vi "Function_queue receiver.vi"(8 "error in (no error)":errorcluster, 9 "Clone Name":string, 11 "Queue in":refnum<queue>) -> (0 "error out":errorcluster, 1 "Filename":string, 3 "Queue out":refnum<queue>, 4 "message":string, 5 "Stop":bool)   [LabVIEW 2022 SP3]
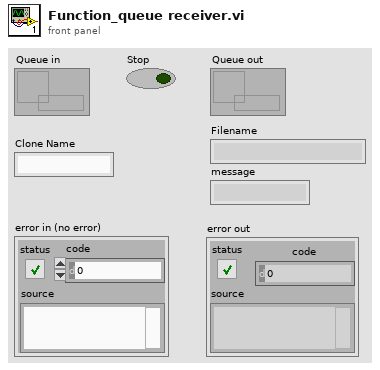
[diagram p1: front panel]
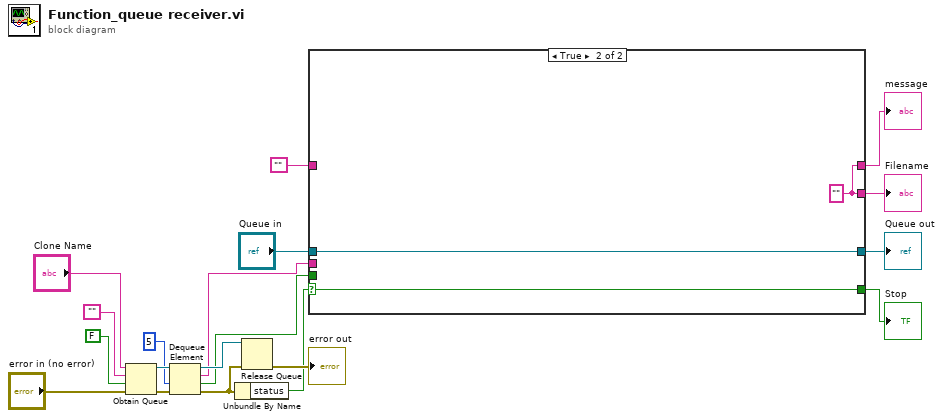
[diagram p0: block diagram]
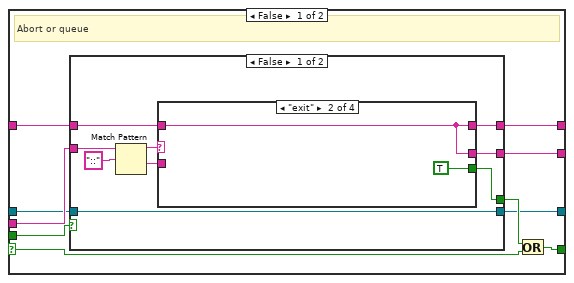
[diagram p2: hidden frame]
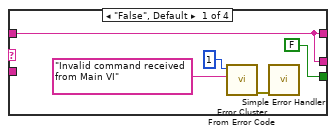
[diagram p3: hidden frame]
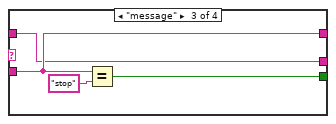
[diagram p4: hidden frame]
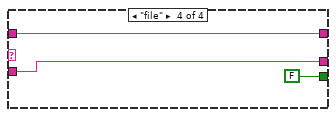
[diagram p5: hidden frame]
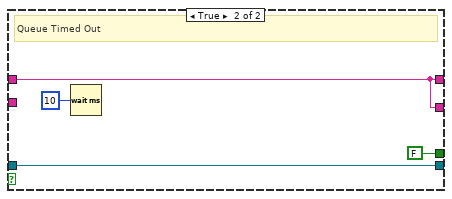
[diagram p6: hidden frame]
diagram:
  n1 = Obtain Queue(name (unnamed)="Clone Name", element data type="", create if not found? (T)=FALSE, error in (no error)="error in (no error)") -> (queue out=w8:refnum<queue>, error out=w9:errorcluster)  [unwired: 1 in, 1 out]
  n2 = Dequeue Element(queue=w8, timeout in ms (-1)=5, error in (no error)=w9) -> (queue out=w12:refnum<queue>, element=w6:string, timed out?=w5:bool, error out=w13:errorcluster)
  n3 = Unbundle By Name(w13) -> ("status"=w7:bool)
  n4 = Release Queue(queue=w12, error in (no error)=w13) -> (error out=→"error out":errorcluster)  [unwired: 1 in, 2 out]
  n5 = case shown="True" w7 {
    selector: w7 -> [w26 w59]
    tunnel: [w25 w59] -> w14
    tunnel: "Queue in" -> [w24 w58]
    tunnel: [w23 w58] -> w3
    tunnel: w5 -> [w29 _]
    tunnel: w6 -> [w28 _]
    tunnel: [w22 w57] -> w18
    tunnel: [w21 w57] -> w19
    tunnel: "" -> [w20 _]
    frame False {
      # "Abort or queue"
      n6 = case shown="False" w29 {
        tunnel: w28 -> [w37 _]
        tunnel: [w35 FALSE] -> w27
        tunnel: w24 -> [w34 w56]
        tunnel: [w34 w56] -> w23
        tunnel: [w32 w53] -> w22
        tunnel: [w31 w53] -> w21
        tunnel: w20 -> [w30 w53]
        frame False {
          n7 = Match Pattern(string=w37, regular expression="::") -> (before substring=w38:string, after substring=w33:string)  [unwired: 1 in, 2 out]
          n8 = case shown="\"exit\"" w38 {
            tunnel: [FALSE TRUE w48 FALSE] -> w35
            tunnel: w33 -> [_ _ w47 w51]
            tunnel: [w39 w44 w46 w51] -> w32
            tunnel: [w39 w44 w47 w50] -> w31
            tunnel: w30 -> [w39 w44 w46 w50]
            frame "False", Default {
              n9 = call <vilib>:"Error Cluster From Error Code.vi"("error message (\"\")"="Invalid command received from Main VI" ("error message (\"\")"), "error code (0)"=1) -> ("error out"=w41:errorcluster)  [unwired: 7 in]
              n10 = call <vilib>:"Simple Error Handler.vi"("error in (no error)"=w41) -> ()  [unwired: 4 in, 5 out]
            }
            frame "exit" {
            }
            frame "message" {
              n11 = Equal?(x=w47, y="stop") -> (x = y?=w48:bool)
            }
            frame "file" {
            }
          }
        }
        frame True {
          # "Queue Timed Out"
          n12 = Wait (ms)(milliseconds to wait=u32 10) -> ()  [unwired: 1 out]
        }
      }
      n13 = Or(x=w27, y=w26) -> (x .or. y?=w25:bool)
    }
    frame True {
      w57 = ""
    }
  }
  "Filename" <- w18
  "message" <- w19
  "Stop" <- w14
  "Queue out" <- w3
